vi "Execute Function.vi"(8 "error in":errorcluster, 10 "modbus request":refnum<class "Modbus Data Unit.lvclass">, 11 "device data model in":refnum<class "Standard Data Model.lvclass">) -> (0 "error out":errorcluster, 2 "modbus response":refnum<class "Modbus Data Unit.lvclass">, 3 "device data model out":refnum<class "Standard Data Model.lvclass">)   [LabVIEW 2013, in "Modbus Library - Advance.lvlib" / "Standard Data Model.lvclass"]
doc: "This function is responsible for deciding what code to execute when a specific function is called."
uses:
  Standard Data Model.lvclass
  Modbus Data Unit/Modbus Data Unit.lvclass
  Modbus Data Unit/Modbus Data Unit.lvclass/Modbus Data Unit.ctl
  Utility/Bits to Bytes.vi
  Utility/Bytes to Bits.vi
  Utility/U16s to Bytes.vi
  Utility/Bytes to U16s.vi
  Data Model/Validate Device ID Code.vi
  Data Model/Search Object List.vi
  Data Model/Process Objects.vi
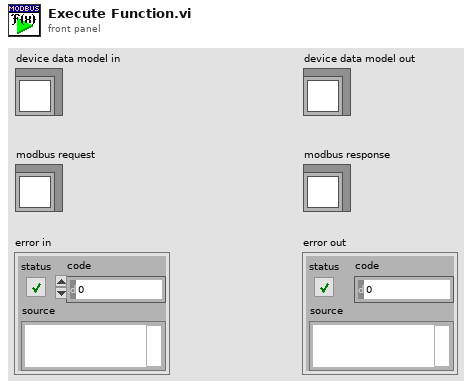
[diagram p1: front panel]
types:
  T1 = typedef "Modbus Library - Advance.lvlib/Modbus Data Unit.lvclass/Function.ctl" = u8
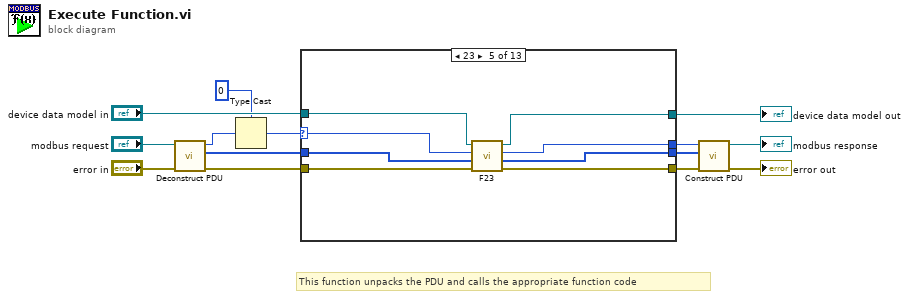
[diagram p0: block diagram]
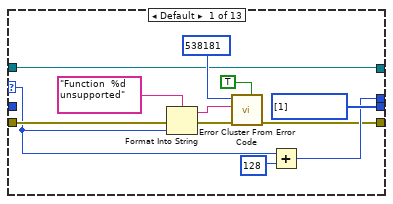
[diagram p2: hidden frame]
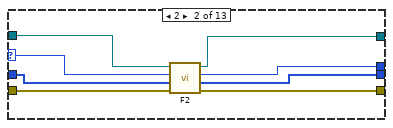
[diagram p3: hidden frame]
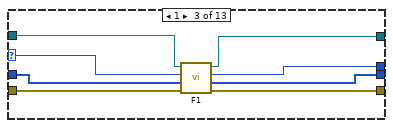
[diagram p4: hidden frame]
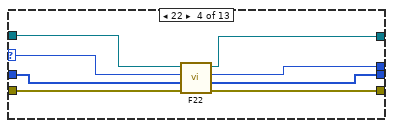
[diagram p5: hidden frame]
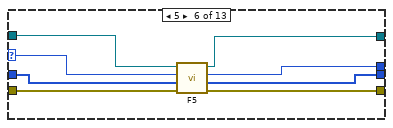
[diagram p6: hidden frame]
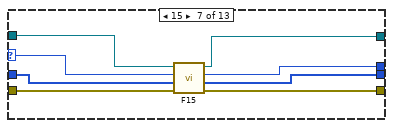
[diagram p7: hidden frame]
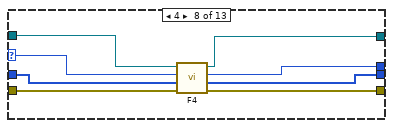
[diagram p8: hidden frame]
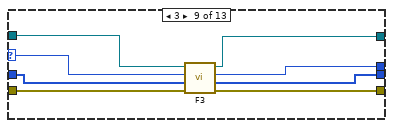
[diagram p9: hidden frame]
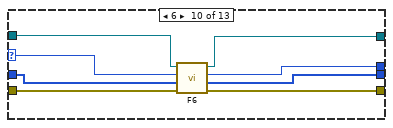
[diagram p10: hidden frame]
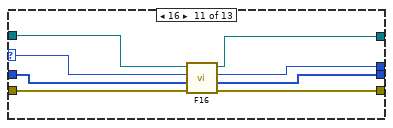
[diagram p11: hidden frame]
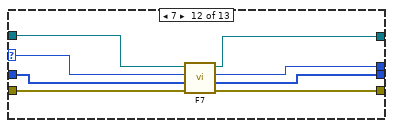
[diagram p12: hidden frame]
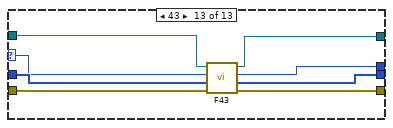
[diagram p13: hidden frame]
diagram:
  # "This function unpacks the PDU and calls the appropriate function code"
  n1 = call "Deconstruct PDU.vi"("error in"="error in", "modbus data unit in"="modbus request") -> ("error out"=w4:errorcluster, "data"=w10:u8[], "Function"=w3:T1)  [unwired: 7 in]
  n2 = Type Cast(type=u8 0, x=w3) -> (*(type *) &x=w2:u8)
  n3 = case shown="23" w2 {
    selector: w2 -> [w15 w33 w39 w47 w55 w62 w73 w77 w89 w96 w101 w112 w115]
    tunnel: "device data model in" -> [w16 w34 w42 w50 w58 w63 w71 w76 w90 w97 w103 w113 w118]
    tunnel: w4 -> [w21 w31 w41 w49 w57 w60 w74 w79 w88 w98 w106 w114 w122]
    tunnel: [w23 w30 w40 w48 w56 w66 w69 w80 w86 w94 w105 w108 w121] -> w9
    tunnel: w10 -> [_ w32 w38 w46 w54 w61 w72 w78 w87 w95 w102 w111 w116]
    tunnel: [w24 w28 w37 w45 w53 w64 w67 w81 w84 w92 w100 w110 w119] -> w7
    tunnel: [u8[] [1] ("Data Return") w29 w36 w44 w52 w65 w68 w82 w85 w93 w99 w109 w120] -> w8
    tunnel: [w16 w27 w35 w43 w51 w59 w70 w75 w83 w91 w104 w107 w117] -> w13
    frame Default {
      n4 = Format Into String(format string="Function  %d unsupported", error in=w21, w15) -> (resulting string=w19:string, error out=w22:errorcluster)  [unwired: 1 in]
      n5 = call <vilib>:"Error Cluster From Error Code.vi"("is warning? (False)"=TRUE, "error in (no error)"=w22, "error message (\"\")"=w19, "error code (0)"=538181) -> ("error out"=w23:errorcluster)  [unwired: 5 in]
      n6 = Add(x=w15, y=u8 128) -> (x+y=w24:u8)
    }
    frame 2 {
      n7 = call "F2.vi"("error in"=w31, "data"=w32, "function"=w33, "device data model in"=w34) -> ("error out"=w30:errorcluster, "data return"=w29:u8[], "function return"=w28:u8, "device data model out"=w27:refnum<class "Standard Data Model.lvclass">)  [unwired: 4 in]
    }
    frame 1 {
      n8 = call "F1.vi"("error in"=w41, "data"=w38, "function"=w39, "device data model in"=w42) -> ("error out"=w40:errorcluster, "data return"=w36:u8[], "function return"=w37:u8, "device data model out"=w35:refnum<class "Standard Data Model.lvclass">)  [unwired: 4 in]
    }
    frame 22 {
      n9 = call "F22.vi"("error in"=w49, "data"=w46, "function"=w47, "device data model in"=w50) -> ("error out"=w48:errorcluster, "data return"=w44:u8[], "function return"=w45:u8, "device data model out"=w43:refnum<class "Standard Data Model.lvclass">)  [unwired: 4 in]
    }
    frame 23 {
      n10 = call "F23.vi"("error in"=w57, "data"=w54, "function"=w55, "device data model in"=w58) -> ("error out"=w56:errorcluster, "data return"=w52:u8[], "function return"=w53:u8, "device data model out"=w51:refnum<class "Standard Data Model.lvclass">)  [unwired: 4 in]
    }
    frame 5 {
      n11 = call "F5.vi"("error in"=w60, "data"=w61, "function"=w62, "device data model in"=w63) -> ("error out"=w66:errorcluster, "data return"=w65:u8[], "function return"=w64:u8, "device data model out"=w59:refnum<class "Standard Data Model.lvclass">)  [unwired: 4 in]
    }
    frame 15 {
      n12 = call "F15.vi"("error in"=w74, "data"=w72, "function"=w73, "device data model in"=w71) -> ("error out"=w69:errorcluster, "data return"=w68:u8[], "function return"=w67:u8, "device data model out"=w70:refnum<class "Standard Data Model.lvclass">)  [unwired: 4 in]
    }
    frame 4 {
      n13 = call "F4.vi"("error in"=w79, "data"=w78, "function"=w77, "device data model in"=w76) -> ("error out"=w80:errorcluster, "data return"=w82:u8[], "function return"=w81:u8, "device data model out"=w75:refnum<class "Standard Data Model.lvclass">)  [unwired: 4 in]
    }
    frame 3 {
      n14 = call "F3.vi"("error in"=w88, "data"=w87, "function"=w89, "device data model in"=w90) -> ("error out"=w86:errorcluster, "data return"=w85:u8[], "function return"=w84:u8, "device data model out"=w83:refnum<class "Standard Data Model.lvclass">)  [unwired: 4 in]
    }
    frame 6 {
      n15 = call "F6.vi"("error in"=w98, "data"=w95, "function"=w96, "device data model in"=w97) -> ("error out"=w94:errorcluster, "data return"=w93:u8[], "function return"=w92:u8, "device data model out"=w91:refnum<class "Standard Data Model.lvclass">)  [unwired: 4 in]
    }
    frame 16 {
      n16 = call "F16.vi"("error in"=w106, "data"=w102, "function"=w101, "device data model in"=w103) -> ("error out"=w105:errorcluster, "data return"=w99:u8[], "function return"=w100:u8, "device data model out"=w104:refnum<class "Standard Data Model.lvclass">)  [unwired: 4 in]
    }
    frame 7 {
      n17 = call "F7.vi"("error in"=w114, "data"=w111, "function"=w112, "device data model in"=w113) -> ("error out"=w108:errorcluster, "data return"=w109:u8[], "function return"=w110:u8, "device data model out"=w107:refnum<class "Standard Data Model.lvclass">)  [unwired: 4 in]
    }
    frame 43 {
      n18 = call "F43.vi"("error in"=w122, "data"=w116, "function"=w115, "device data model in"=w118) -> ("error out"=w121:errorcluster, "data return"=w120:u8[], "function return"=w119:u8, "device data model out"=w117:refnum<class "Standard Data Model.lvclass">)  [unwired: 4 in]
    }
  }
  "device data model out" <- w13
  n19 = call "Construct PDU.vi"("error in"=w9, "data"=w8, "Function"=w7) -> ("error out"=→"error out":errorcluster, "modbus data unit out"=→"modbus response":refnum<class "Modbus Data Unit.lvclass">)  [unwired: 7 in]
